vi "previous_call_no.vi"() -> (3 "Previous Call No.":string)   [LabVIEW 2023]
uses:
  <vilib>/addons/database/Auxilliary.llb/DB Tools Cursor Type.ctl
  <vilib>/addons/database/Connection.llb/DB Tools Open Connec (Path).vi
  <vilib>/addons/database/Connection.llb/Conn Execute.vi
  <vilib>/addons/database/Recordset.llb/Rec Fetch String Data (R).vi
  <vilib>/addons/database/Recordset.llb/Rec Destroy - Connection.vi
  <vilib>/addons/database/NI_Database_API.lvlib
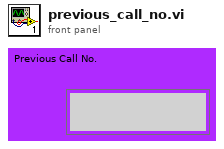
[diagram p1: front panel]
types:
  T1 = typedef "NI_Database_API.lvlib/DB Tools Cursor Type.ctl" = enum16{"forward-only", "keyset", "dynamic", "static"}
  T2 = typedef "NI_Database_API.lvlib/Conn ObjectReference.ctl" = refnum<k1>
  T3 = typedef "NI_Database_API.lvlib/Rec ObjectReference.ctl" = refnum<k1>
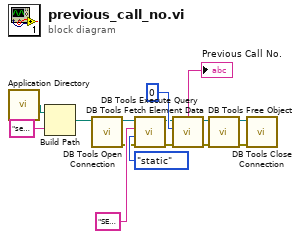
[diagram p0: block diagram]
diagram:
  n1 = call <vilib>:"Application Directory.vi"() -> ("Application Directory"=w1:path)
  n2 = Build Path(base path=w1, name or relative path="service_calls_entries.udl") -> (appended path=w3:path)
  n3 = call-poly <vilib>:"DB Tools Open Connection.vi"("connection information"=w3) -> ("error out"=w5:errorcluster, "connection reference"=w4:T2)  [unwired: 7 in]
  n4 = call-poly <vilib>:"DB Tools Execute Query.vi"("error in (no error)"=w5, "cursor type"=DB_Tools_Cursor_Type."static", "SQL query"="SELECT TOP 1 Asset_No FROM Service_Calls_Entry ORDER BY Asset_No DESC;", "connection reference"=w4) -> ("error out"=w8:errorcluster, "recordset reference"=w9:T3)  [unwired: 4 in]
  n5 = call-poly <vilib>:"DB Tools Fetch Element Data.vi"("error in (no error)"=w8, "column index"=0, "recordset reference"=w9) -> ("error out"=w12:errorcluster, "data"=→"Previous Call No.":string, "recordset reference out"=w13:T3)  [unwired: 4 in]
  n6 = call-poly <vilib>:"DB Tools Free Object.vi"("error in (no error)"=w12, "recordset reference"=w13) -> ("error out"=w14:errorcluster, "connection reference"=w15:T2)  [unwired: 8 in]
  n7 = call <vilib>:"DB Tools Close Connection.vi"("error in (no error)"=w14, "connection reference"=w15) -> ()  [unwired: 5 in, 1 out]
